vi "Empty Strategies Map.vi"() -> (2 "Ephemeral Strategies":map{string, refnum<class "BananaPeel.lvclass">}(c390))   [LabVIEW 2021, in "Bananas.lvlib"]
uses:
  Bananas.lvlib
  BananaPeel/BananaPeel.lvclass
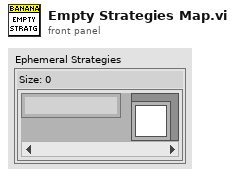
[diagram p1: front panel]
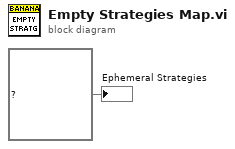
[diagram p0: block diagram]
diagram:
  "Ephemeral Strategies" <- map{string, refnum<class "BananaPeel.lvclass">} {} ("Ephemeral Strategies")
